vi "MainHost.vi"() -> ()   [LabVIEW 2017]
uses:
  TypeDefs/UDPLoopState.ctl
  TypeDefs/UDPListenFGVCtrl.ctl
  TypeDefs/dataFGVState.ctl
  TypeDefs/dataIn.ctl
  TypeDefs/starState.ctl
  TypeDefs/basicFGVControl.ctl
  TypeDefs/starFGVControl.ctl
panel:
  in  "stop star":bool
  in  "start star":bool
  in  "stop":bool
  out "Graph":cluster{dbl[], dbl[]}[](graph)
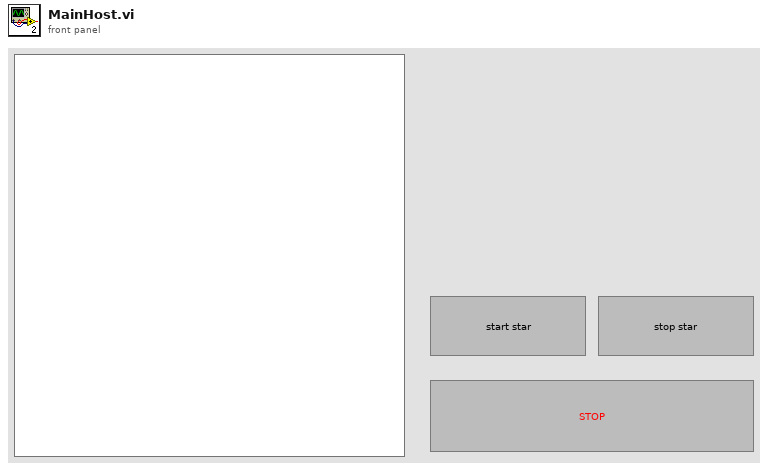
[diagram p1: front panel]
types:
  T1 = typedef "starState.ctl" = enum16{"wait", "1", "2", "3", "4", "5", "end"}
  T2 = typedef "UDPLoopState.ctl" = enum16{"init", "run", "end"}
  T3 = typedef "basicFGVControl.ctl" = enum16{"get", "set"}
  T4 = typedef "starFGVControl.ctl" = enum16{"getAll", "setStop", "setStart"}
  T5 = typedef "dataFGVState.ctl" = enum16{"init", "write data out", "read data out", "write data in", "read data in"}
  T6 = typedef "dataOut.ctl" = cluster{"X0pos":dbl, "Y0pos":dbl, "Z0pos":dbl, "Fx":dbl, "Fy":dbl, "Fz":dbl, "Encoder1":i32, "Encoder2":i32, "Pot1":dbl, "Pot2":dbl, "Theta0":dbl, "Theta1":dbl, "X1pos":dbl, "Y1pos":dbl, "Z1pos":dbl, "X2pos":dbl, "Y2pos":dbl, "Z2pos":dbl, "ErrorOccurred":bool}
  T7 = typedef "UDPListenFGVCtrl.ctl" = enum16{"Read", "Write"}
  T8 = typedef "dataIn.ctl" = cluster{"Xtarget":dbl, "Ytarget":dbl, "Ztarget":dbl, "X_Attractor1":dbl, "Y_Attractor1":dbl, "Z_Attractor1":dbl, "X_Attractor2":dbl, "Y_Attractor2":dbl, "Z_Attractor2":dbl, "Traj_Flag":bool, "DeadZone":dbl, "Assistance":bool, "Shutdown":bool, "AssistanceLevel":dbl}
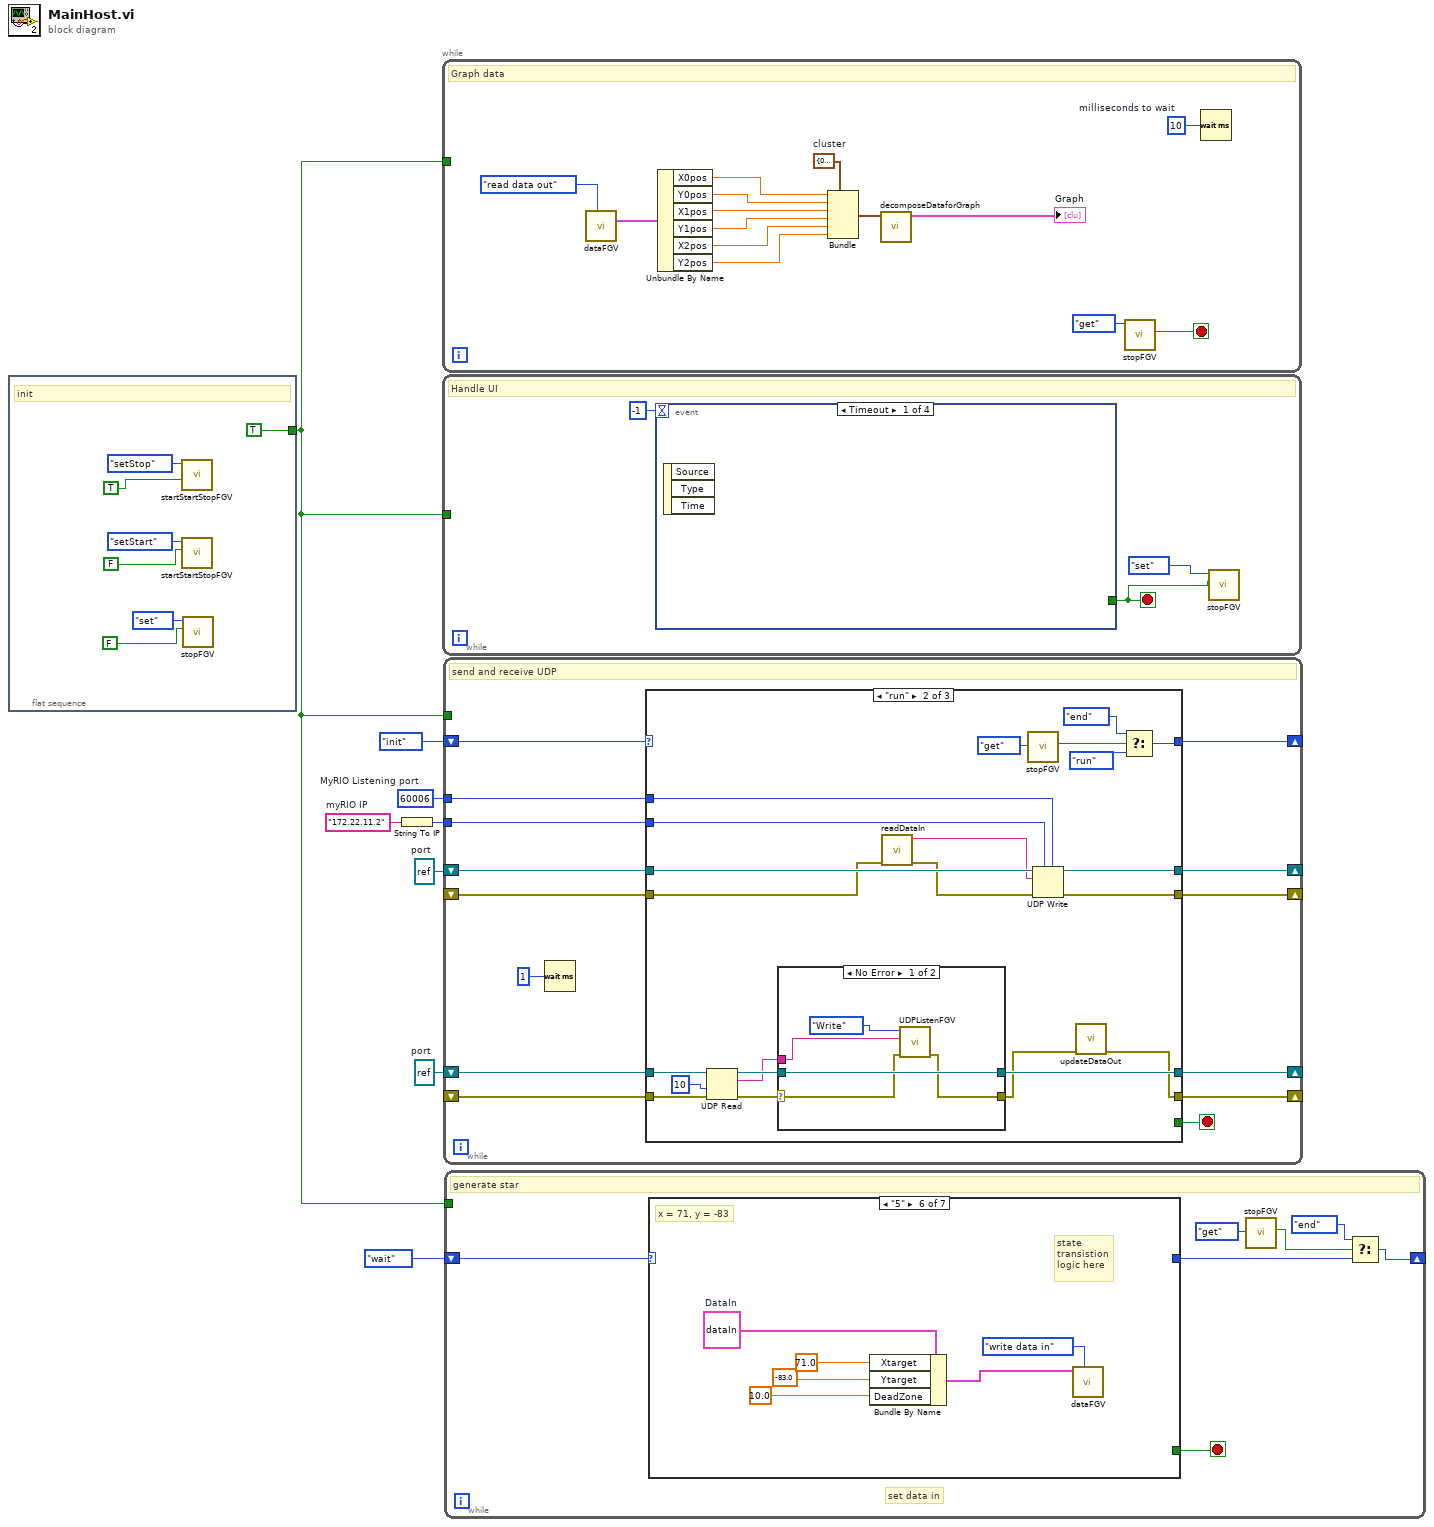
[diagram p0: block diagram]
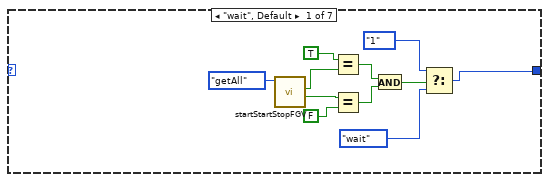
[diagram p2: hidden frame]
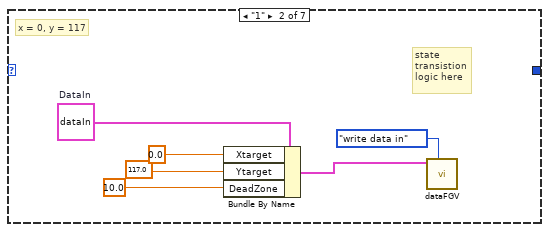
[diagram p3: hidden frame]
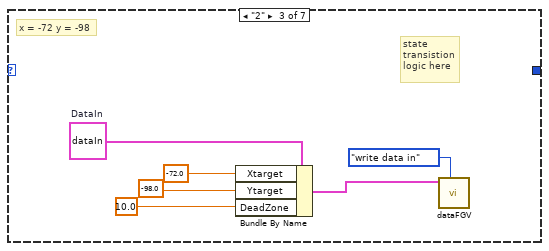
[diagram p4: hidden frame]
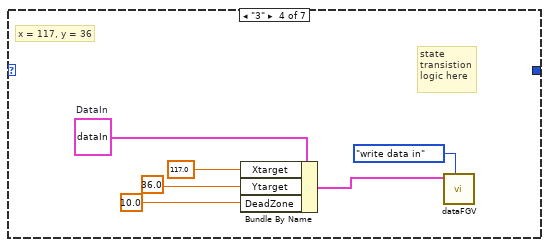
[diagram p5: hidden frame]
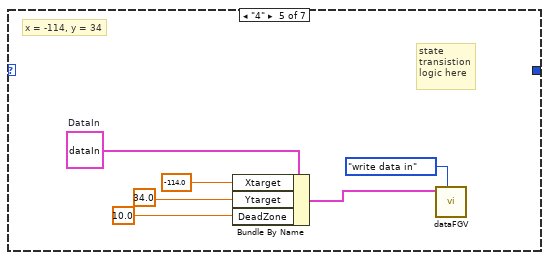
[diagram p6: hidden frame]
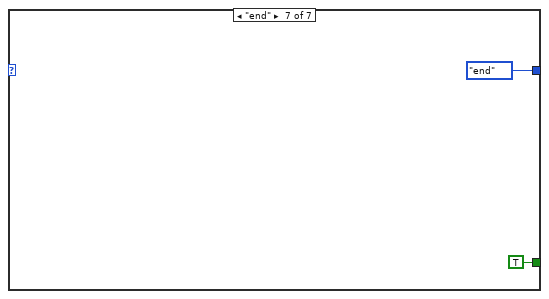
[diagram p7: hidden frame]
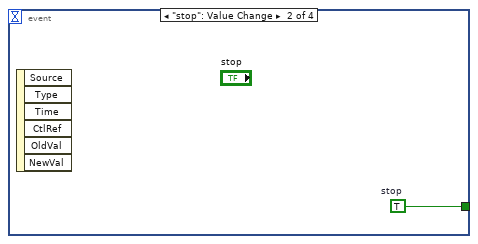
[diagram p8: hidden frame]
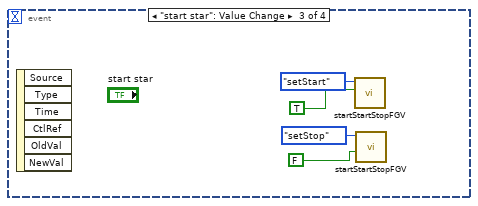
[diagram p9: hidden frame]
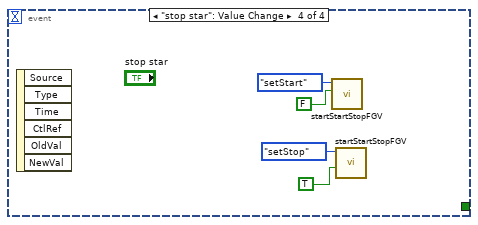
[diagram p10: hidden frame]
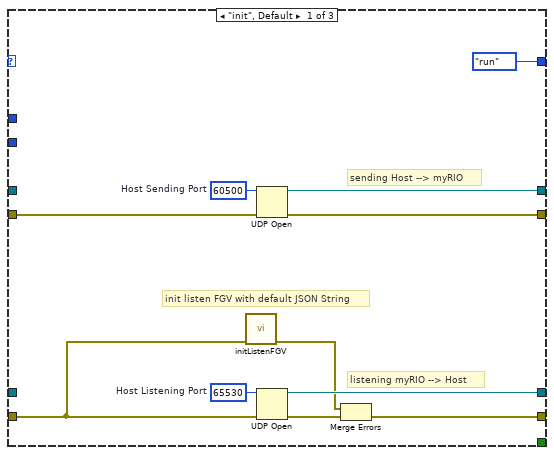
[diagram p11: hidden frame]
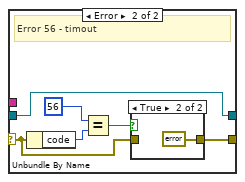
[diagram p12: hidden frame]
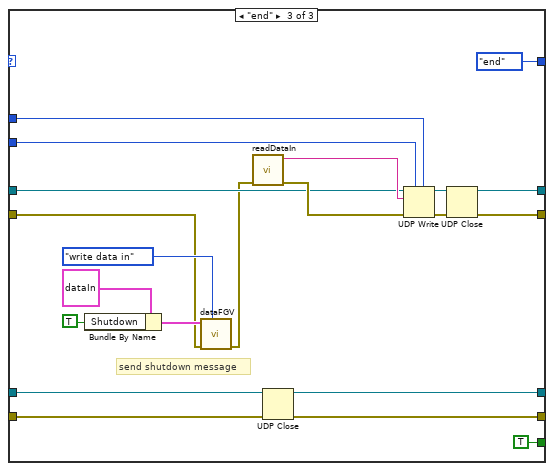
[diagram p14: hidden frame]
diagram:
  w5 = "172.22.11.2"  # myRIO IP
  w4 = u16 60006  # MyRIO Listening port
  w6 = refnum<k16> refnum  # port
  w7 = refnum<k16> refnum  # port
  n1 = flat-sequence {
    tunnel: [TRUE ("stop?")] -> w1
    frame #0 {
      # "init"
      n2 = call "startStartStopFGV.vi"("stop"=TRUE ("stop?"), "Enum"=starFGVControl."setStop") -> ()  [unwired: 8 in, 2 out]
      n3 = call "startStartStopFGV.vi"("start"=FALSE ("stop?"), "Enum"=starFGVControl."setStart") -> ()  [unwired: 8 in, 2 out]
      n4 = call "stopFGV.vi"("stop?"=FALSE, "Enum"=basicFGVControl."set") -> ()  [unwired: 9 in, 1 out]
    }
  }
  n5 = String To IP(1:w5) -> (0:w3:u32)
  n6 = while {
    tunnel: w1 -> [_]
    stop <- w16 stop-if-true
    w18 = u32 10  # milliseconds to wait
    w28 = cluster{dbl, dbl, dbl, dbl, dbl, dbl} {0.0, 0.0, 0.0, 0.0, 0.0, 0.0}  # cluster
    # "Graph data"
    n7 = call "dataFGV.vi"("Enum"=dataFGVState."read data out") -> ("DataOut"=w20:T6)  [unwired: 8 in, 2 out]
    n8 = Unbundle By Name(w20) -> ("X0pos"=w26:dbl, "Y0pos"=w25:dbl, "X1pos"=w24:dbl, "Y1pos"=w23:dbl, "X2pos"=w22:dbl, "Y2pos"=w21:dbl)
    n9 = Bundle(cluster=w28, w26, w25, w24, w23, w22, w21) -> (w27:cluster{dbl, dbl, dbl, dbl, dbl, dbl})
    n10 = call "decomposeDataforGraph.vi"("cluster"=w27) -> ("Array"=→"Graph":cluster{dbl[], dbl[]}[])  [unwired: 10 in]
    n11 = call "stopFGV.vi"("Enum"=basicFGVControl."get") -> ("stop?"=w16:bool)  [unwired: 10 in]
    n12 = Wait (ms)(milliseconds to wait=w18) -> ()  [unwired: 1 out]
  }
  n13 = while {
    tunnel: w1 -> [_]
    stop <- w30 stop-if-true
    # "Handle UI"
    n14 = event shown="[0] Timeout" {
      selector: _ -> [_ _ _ _]
      dyn-events: _ -> [_ _ _ _]
      timeout: -1 -> [_ _ _ _]
      tunnel: [_ w33 _ _] -> w30
      event Timeout {
        n15 = event-data() -> ()  [unwired: 1 in, 3 out]
      }
      event "stop": Value Change {
        w33 = TRUE  # stop
        n16 = event-data() -> ()  [unwired: 1 in, 6 out]
      }
      event "start star": Value Change {
        n17 = event-data() -> ()  [unwired: 1 in, 6 out]
        n18 = call "startStartStopFGV.vi"("start"=TRUE, "Enum"=starFGVControl."setStart") -> ()  [unwired: 8 in, 2 out]
        n19 = call "startStartStopFGV.vi"("stop"=FALSE, "Enum"=starFGVControl."setStop") -> ()  [unwired: 8 in, 2 out]
      }
      event "stop star": Value Change {
        n20 = event-data() -> ()  [unwired: 1 in, 6 out]
        n21 = call "startStartStopFGV.vi"("start"=FALSE, "Enum"=starFGVControl."setStart") -> ()  [unwired: 8 in, 2 out]
        n22 = call "startStartStopFGV.vi"("stop"=TRUE, "Enum"=starFGVControl."setStop") -> ()  [unwired: 8 in, 2 out]
      }
    }
    n23 = call "stopFGV.vi"("stop?"=w30, "Enum"=basicFGVControl."set") -> ()  [unwired: 9 in, 1 out]
  }
  n24 = while {
    shift-right: [w42] -> _
    shift-left: UDPLoopState."init" -> [w55]
    shift-right: [w53] -> _
    shift-left: w7 -> [w48]
    shift-right: [w52] -> _
    shift-left: _ -> [w51]
    shift-right: [w50] -> _
    shift-left: w6 -> [w46]
    shift-right: [w49] -> _
    shift-left: _ -> [w47]
    tunnel: w4 -> [w45]
    tunnel: w3 -> [w44]
    tunnel: w1 -> [_]
    stop <- w54 stop-if-true
    # "send and receive UDP"
    n25 = Wait (ms)(milliseconds to wait=u32 1) -> ()  [unwired: 1 out]
    n26 = case shown="\"run\"" w55 {
      tunnel: [_ _ TRUE] -> w54
      tunnel: [w65 w80 w121] -> w53
      tunnel: [w64 w81 w120] -> w52
      tunnel: w51 -> [w63 w72 w103]
      tunnel: [w61 w82 w117] -> w50
      tunnel: [w58 w75 w116] -> w49
      tunnel: w48 -> [_ w79 w112]
      tunnel: w47 -> [w60 w83 w118]
      tunnel: w46 -> [_ w84 w119]
      tunnel: w45 -> [_ w78 w108]
      tunnel: w44 -> [_ w77 w111]
      tunnel: [UDPLoopState."run" w67 UDPLoopState."end"] -> w42
      frame "init", Default {
        w62 = u16 65530  # Host Listening Port
        w66 = u16 60500  # Host Sending Port
        # "init listen FGV with default JSON String"
        # "listening myRIO --> Host"
        # "sending Host --> myRIO"
        n27 = call "initListenFGV.vi"("error in (no error)"=w60) -> ("error out"=w57:errorcluster)  [unwired: 10 in]
        n28 = UDP Open(8:w63, 11:w66) -> (port=w65:refnum<k16>, 0:w64:errorcluster)  [unwired: 3 in, 1 out]
        n29 = UDP Open(8:w60, 11:w62) -> (port=w61:refnum<k16>, 0:w59:errorcluster)  [unwired: 3 in, 1 out]
        n30 = Merge Errors(w57, w59) -> (w58:errorcluster)
      }
      frame "run" {
        n31 = UDP Read(connection ID=w84, timeout ms (25000)=10, 8:w83) -> (data out=w85:string, error out=w87:errorcluster, 3:w86:refnum<k16>)  [unwired: 1 in, 2 out]
        n32 = case shown="No Error" w87 {
          selector: w87 -> [w92 w95]
          tunnel: w86 -> [w93 w94]
          tunnel: w85 -> [w90 _]
          tunnel: [w91 w96] -> w76
          tunnel: [w93 w94] -> w82
          frame No Error {
            n33 = call "UDPListenFGV.vi"("error in (no error)"=w92, "Write Data"=w90, "Enum"=UDPListenFGVCtrl."Write") -> ("error out"=w91:errorcluster)  [unwired: 7 in, 1 out]
          }
          frame Error {
            # "Error 56 - timout"
            n34 = Unbundle By Name(w95) -> ("code"=w99:i32)
            n35 = Equal?(x=56, y=w99) -> (x = y?=w97:bool)
            n36 = case shown="True" w97 {
              tunnel: [w100 errorcluster {"status"=FALSE, "code"=0, "source"=""} ("error constant")] -> w96
              tunnel: w95 -> [w100 _]
              frame False {
              }
              frame True {
              }
            }
          }
        }
        n37 = call "readDataIn.vi"("error in (no error)"=w72) -> ("error out"=w73:errorcluster, "JSON string"=w74:string)  [unwired: 9 in]
        n38 = call "stopFGV.vi"("Enum"=basicFGVControl."get") -> ("stop?"=w70:bool)  [unwired: 10 in]
        n39 = UDP Write(address=w77, port or service name=w78, connection ID=w79, data in=w74, 8:w73) -> (error out=w81:errorcluster, 3:w80:refnum<k16>)  [unwired: 1 in]
        n40 = call "updateDataOut.vi"("error in (no error)"=w76) -> ("error out"=w75:errorcluster)  [unwired: 10 in]
        n41 = Select(t=UDPLoopState."end", s=w70, f=UDPLoopState."run") -> (s? t:f=w67:T2)
      }
      frame "end" {
        # "send shutdown message"
        n42 = Bundle By Name(cluster=T8 {"Xtarget"=0.0, "Ytarget"=0.0, "Ztarget"=0.0, "X_Attractor1"=0.0, "Y_Attractor1"=0.0, "Z_Attractor1"=0.0, "X_Attractor2"=0.0, "Y_Attractor2"=0.0, "Z_Attractor2"=0.0, "Traj_Flag"=FALSE, "DeadZone"=0.0, "Assistance"=FALSE, "Shutdown"=FALSE, "AssistanceLevel"=0.0} ("DataIn"), "Shutdown"=TRUE) -> (w104:T8)
        n43 = call "dataFGV.vi"("Enum"=dataFGVState."write data in", "error in (no error)"=w103, "DataIn"=w104) -> ("error out"=w102:errorcluster)  [unwired: 6 in, 2 out]
        n44 = call "readDataIn.vi"("error in (no error)"=w102) -> ("error out"=w113:errorcluster, "JSON string"=w114:string)  [unwired: 9 in]
        n45 = UDP Close(connection ID=w119, 8:w118) -> (connection ID out=w117:refnum<k16>, error out=w116:errorcluster)
        n46 = UDP Write(address=w111, port or service name=w108, connection ID=w112, data in=w114, 8:w113) -> (error out=w109:errorcluster, 3:w110:refnum<k16>)  [unwired: 1 in]
        n47 = UDP Close(connection ID=w110, 8:w109) -> (connection ID out=w121:refnum<k16>, error out=w120:errorcluster)
      }
    }
  }
  n48 = while {
    shift-right: [w124] -> _
    shift-left: starState."wait" -> [w129]
    tunnel: w1 -> [_]
    stop <- w128 stop-if-true
    # "set data in"
    # "generate star"
    n49 = case shown="\"5\"" w129 {
      tunnel: [_ _ _ _ _ _ TRUE] -> w128
      tunnel: [w130 _ _ _ _ _ starState."end"] -> w125
      frame "wait", Default {
        n50 = call "startStartStopFGV.vi"("Enum"=starFGVControl."getAll") -> ("stop"=w137:bool, "start"=w139:bool)  [unwired: 9 in]
        n51 = Equal?(x=TRUE, y=w139) -> (x = y?=w134:bool)
        n52 = Equal?(x=w137, y=FALSE) -> (x = y?=w135:bool)
        n53 = And(x=w134, y=w135) -> (x .and. y?=w133:bool)
        n54 = Select(t=starState."1", s=w133, f=starState."wait") -> (s? t:f=w130:T1)
      }
      frame "1" {
        w145 = T8 {"Xtarget"=0.0, "Ytarget"=0.0, "Ztarget"=0.0, "X_Attractor1"=0.0, "Y_Attractor1"=0.0, "Z_Attractor1"=0.0, "X_Attractor2"=0.0, "Y_Attractor2"=0.0, "Z_Attractor2"=0.0, "Traj_Flag"=FALSE, "DeadZone"=0.0, "Assistance"=FALSE, "Shutdown"=FALSE, "AssistanceLevel"=0.0}  # DataIn
        # "x = 0, y = 117"
        # "state\ntransistion\nlogic here"
        n55 = Bundle By Name(cluster=w145, "Xtarget"=0.0, "Ytarget"=117.0, "DeadZone"=10.0) -> (w144:T8)
        n56 = call "dataFGV.vi"("Enum"=dataFGVState."write data in", "DataIn"=w144) -> ()  [unwired: 7 in, 3 out]
      }
      frame "2" {
        w151 = T8 {"Xtarget"=0.0, "Ytarget"=0.0, "Ztarget"=0.0, "X_Attractor1"=0.0, "Y_Attractor1"=0.0, "Z_Attractor1"=0.0, "X_Attractor2"=0.0, "Y_Attractor2"=0.0, "Z_Attractor2"=0.0, "Traj_Flag"=FALSE, "DeadZone"=0.0, "Assistance"=FALSE, "Shutdown"=FALSE, "AssistanceLevel"=0.0}  # DataIn
        # "x = -72 y = -98"
        # "state\ntransistion\nlogic here"
        n57 = Bundle By Name(cluster=w151, "Xtarget"=-72.0, "Ytarget"=-98.0, "DeadZone"=10.0) -> (w150:T8)
        n58 = call "dataFGV.vi"("Enum"=dataFGVState."write data in", "DataIn"=w150) -> ()  [unwired: 7 in, 3 out]
      }
      frame "3" {
        w157 = T8 {"Xtarget"=0.0, "Ytarget"=0.0, "Ztarget"=0.0, "X_Attractor1"=0.0, "Y_Attractor1"=0.0, "Z_Attractor1"=0.0, "X_Attractor2"=0.0, "Y_Attractor2"=0.0, "Z_Attractor2"=0.0, "Traj_Flag"=FALSE, "DeadZone"=0.0, "Assistance"=FALSE, "Shutdown"=FALSE, "AssistanceLevel"=0.0}  # DataIn
        # "x = 117, y = 36"
        # "state\ntransistion\nlogic here"
        n59 = Bundle By Name(cluster=w157, "Xtarget"=117.0, "Ytarget"=36.0, "DeadZone"=10.0) -> (w156:T8)
        n60 = call "dataFGV.vi"("Enum"=dataFGVState."write data in", "DataIn"=w156) -> ()  [unwired: 7 in, 3 out]
      }
      frame "4" {
        w163 = T8 {"Xtarget"=0.0, "Ytarget"=0.0, "Ztarget"=0.0, "X_Attractor1"=0.0, "Y_Attractor1"=0.0, "Z_Attractor1"=0.0, "X_Attractor2"=0.0, "Y_Attractor2"=0.0, "Z_Attractor2"=0.0, "Traj_Flag"=FALSE, "DeadZone"=0.0, "Assistance"=FALSE, "Shutdown"=FALSE, "AssistanceLevel"=0.0}  # DataIn
        # "x = -114, y = 34"
        # "state\ntransistion\nlogic here"
        n61 = Bundle By Name(cluster=w163, "Xtarget"=-114.0, "Ytarget"=34.0, "DeadZone"=10.0) -> (w162:T8)
        n62 = call "dataFGV.vi"("Enum"=dataFGVState."write data in", "DataIn"=w162) -> ()  [unwired: 7 in, 3 out]
      }
      frame "5" {
        w169 = T8 {"Xtarget"=0.0, "Ytarget"=0.0, "Ztarget"=0.0, "X_Attractor1"=0.0, "Y_Attractor1"=0.0, "Z_Attractor1"=0.0, "X_Attractor2"=0.0, "Y_Attractor2"=0.0, "Z_Attractor2"=0.0, "Traj_Flag"=FALSE, "DeadZone"=0.0, "Assistance"=FALSE, "Shutdown"=FALSE, "AssistanceLevel"=0.0}  # DataIn
        # "x = 71, y = -83"
        # "state\ntransistion\nlogic here"
        n63 = Bundle By Name(cluster=w169, "Xtarget"=71.0, "Ytarget"=-83.0, "DeadZone"=10.0) -> (w168:T8)
        n64 = call "dataFGV.vi"("Enum"=dataFGVState."write data in", "DataIn"=w168) -> ()  [unwired: 7 in, 3 out]
      }
      frame "end" {
      }
    }
    n65 = call "stopFGV.vi"("Enum"=basicFGVControl."get") -> ("stop?"=w126:bool)  [unwired: 10 in]
    n66 = Select(t=starState."end", s=w126, f=w125) -> (s? t:f=w124:T1)
  }
